vi "parse_poseWithCovariance.vi"(4 "error in (no error)":errorcluster, 7 "msg in":string) -> (0 "error out":errorcluster, 2 "PoseCovariance":T1, 3 "msg out":string)   [LabVIEW 2012]
doc: "Parses a message into a pose with covariance"
uses:
  std_msgs/subs/parse_float64_scalar.vi
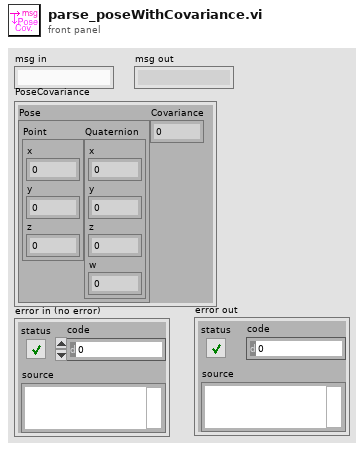
[diagram p1: front panel]
types:
  T1 = cluster{"Pose":cluster{"Point":cluster{"x":dbl, "y":dbl, "z":dbl}, "Quaternion":cluster{"x":dbl, "y":dbl, "z":dbl, "w":dbl}}, "Covariance":dbl}
  T2 = cluster{"Point":cluster{"x":dbl, "y":dbl, "z":dbl}, "Quaternion":cluster{"x":dbl, "y":dbl, "z":dbl, "w":dbl}}
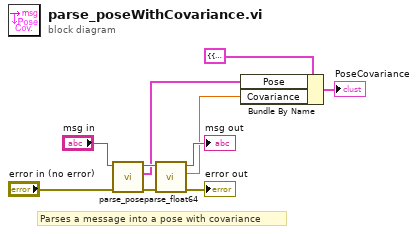
[diagram p0: block diagram]
diagram:
  # "Parses a message into a pose with covariance"
  n1 = call "parse_pose.vi"("error in"="error in (no error)", "msg in"="msg in") -> ("error out"=w8:errorcluster, "Pose"=w2:T2, "msg out"=w7:string)  [unwired: 3 in]
  n2 = call-poly "parse_float64.vi"("error in"=w8, "msg in"=w7) -> ("error out"=→"error out":errorcluster, "number"=w1:dbl, "msg out"=→"msg out":string)  [unwired: 3 in]
  n3 = Bundle By Name(cluster=T1 {"Pose"={"Point"={"x"=0.0, "y"=0.0, "z"=0.0}, "Quaternion"={"x"=0.0, "y"=0.0, "z"=0.0, "w"=0.0}}, "Covariance"=0.0} ("PoseCovariance"), "Pose"=w2, "Covariance"=w1) -> (→"PoseCovariance":T1)
